vi "BW Calc Wrapper.vi"(2 "Data Value Reference in":refnum<data-value>) -> (3 "MB/s":dbl, 4 "Data Value Reference out":refnum<data-value>)   [LabVIEW 2021, in "DecodetoImage.lvlib"]
uses:
  DecodetoImage.lvlib
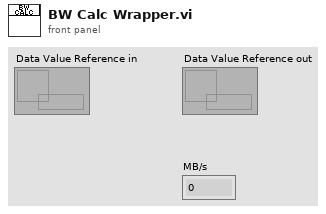
[diagram p1: front panel]
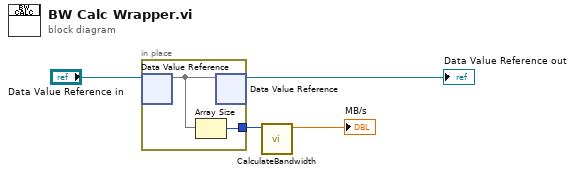
[diagram p0: block diagram]
diagram:
  n1 = in-place {
    in-place-border: [w5] -> w3
    n2 = in-place-dvr #1("Data Value Reference in") -> (w6:u8[])  [unwired: 1 out]
    n3 = Array Size(array=w6) -> (size(s)=w5:i32)
    n4 = in-place-dvr #1(w6) -> (→"Data Value Reference out":refnum<data-value>)  [unwired: 1 out]
  }
  n5 = call "CalculateBandwidth.vi"("New Bytes Transferred"=w3) -> ("MB/s"=→"MB/s":dbl)  [unwired: 10 in]
